vi "Prime BSI R3 Get Set ROI.vi"(0 "Prime Notifier":refnum<notifier>, 7 "IDS Actions":T2, 11 "Camera Handle":u32, 13 "Image Ref":T1) -> (4 "Prime Notifier (Dup)":refnum<notifier>, 15 "Error":errorcluster)   [LabVIEW 2016]
uses:
  Prime Controls/Prime Notifier Element.ctl
  Prime Controls/Prime Actions.ctl
  Prime Controls/Prime Parameters.ctl
  Prime Controls/Prime Parameter List.ctl
  Prime Controls/Prime ROI.ctl
  <vilib>/vision/Image Controls.llb/IMAQ Image.ctl
  Prime Controls/Prime IMAQ Key Info.ctl
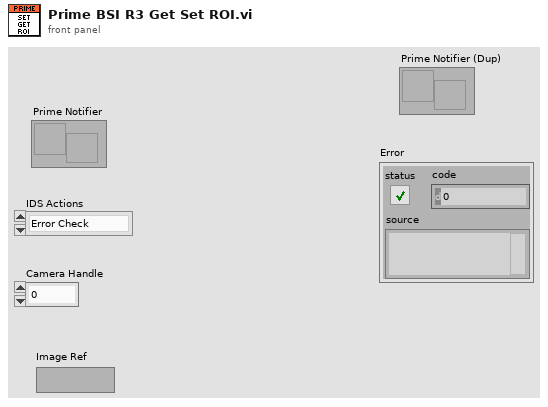
[diagram p1: front panel]
types:
  T1 = typedef "IMAQ Image.ctl" = refnum<image>
  T2 = typedef "Prime Actions.ctl" = enum16{"Error Check", "Initialize", "Preview", "Record", "Abort", "Record Settings", "Set Parameter", "Get Parameter", "Set ROI", "Get ROI", "Status", "Quit"}
  T3 = typedef "Prime IMAQ Key Info.ctl" = cluster{"Frame":u32, "Sensor Height":i32, "Sensor Width":i32, "ROI Height":i32, "ROI Width":i32, "ROI Enable?":bool, "Bit per Pixel":u8}
  T4 = typedef "Prime ROI.ctl" = cluster{"X Start":u32, "X End":u32, "X Bin":u32, "Y Start":u32, "Y End":u32, "Y Bin":u32}
  T5 = typedef "Prime Notifier Element.ctl" = cluster{"Prime Actions":T2, "Received?":bool, "Prime Parameter":T6, "Prime ROI":T4, "Running?":bool, "File Path":path, "# of frames":i32, "Image Ref":T1, "Error":errorcluster}
  T6 = typedef "Prime Parameters.ctl" = cluster{"Parameter":T7, "Value":dbl}
  T7 = typedef "Prime Parameter List.ctl" = enum16{"Exposure Time (s)"}
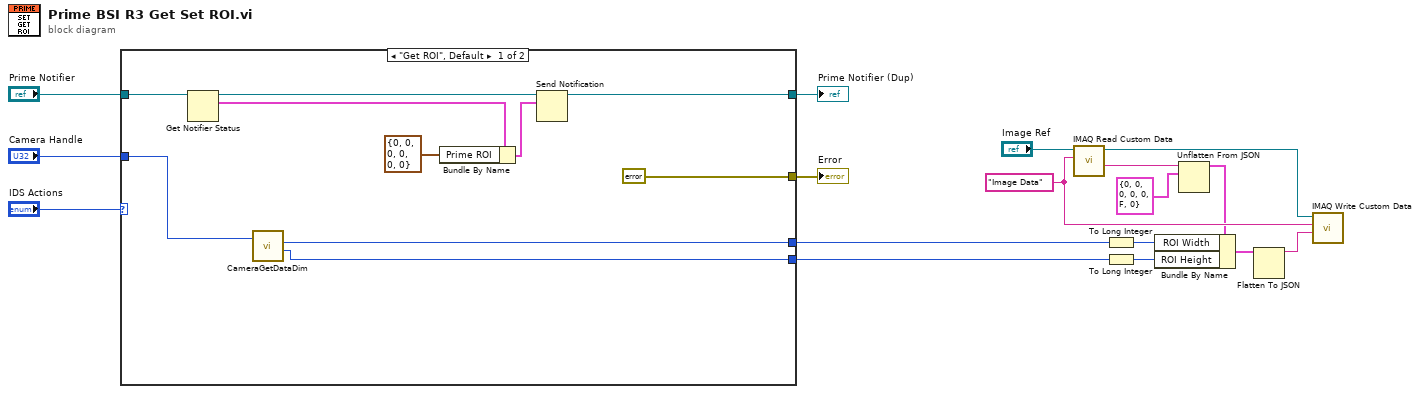
[diagram p0: block diagram]
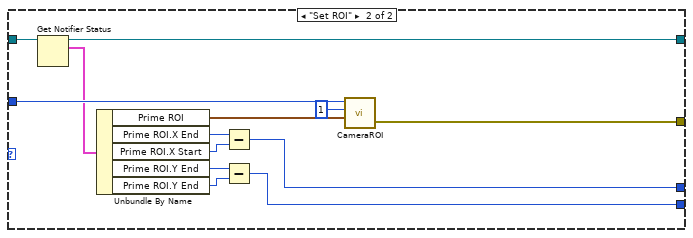
[diagram p2: hidden frame]
diagram:
  w12 = "Image Data" ("Key")
  n1 = case shown="\"Get ROI\", Default" "IDS Actions" {
    tunnel: "Prime Notifier" -> [w27 w38]
    tunnel: [w25 w37] -> w15
    tunnel: "Camera Handle" -> [w20 w40]
    tunnel: [errorcluster {"status"=FALSE, "code"=0, "source"=""} ("error out") w34] -> w13
    tunnel: [w19 w29] -> w1
    tunnel: [w18 w28] -> w2
    frame "Get ROI", Default {
      n2 = Get Notifier Status(notifier=w27) -> (notifier out=w26:refnum<notifier>, current notification=w24:T5)  [unwired: 1 in, 3 out]
      n3 = call <userlib>:"CameraGetDataDim.vi"("Camera Handle"=w20) -> ("Xdim"=w19:u32, "Ydim"=w18:u32)  [unwired: 1 in, 2 out]
      n4 = Bundle By Name(cluster=w24, "Prime ROI"=T4 {"X Start"=0, "X End"=0, "X Bin"=0, "Y Start"=0, "Y End"=0, "Y Bin"=0} ("IDS ROI")) -> (w23:T5)
      n5 = Send Notification(notification=w23, notifier=w26) -> (notifier out=w25:refnum<notifier>)  [unwired: 1 in, 1 out]
    }
    frame "Set ROI" {
      n6 = Get Notifier Status(notifier=w38) -> (notifier out=w37:refnum<notifier>, current notification=w36:T5)  [unwired: 1 in, 3 out]
      n7 = Unbundle By Name(w36) -> ("Prime ROI"=w35:T4, "Prime ROI.X End"=w33:u32, "Prime ROI.X Start"=w32:u32, "Prime ROI.Y End"=w31:u32, "Prime ROI.Y End"=w30:u32)
      n8 = Subtract(x=w33, y=w32) -> (x-y=w29:u32)
      n9 = Subtract(x=w31, y=w30) -> (x-y=w28:u32)
      n10 = call <userlib>:"CameraROI.vi"("ROI Params"=w35, "ROI Index"=u32 1, "Camera Handle"=w40) -> ("error out"=w34:errorcluster)  [unwired: 1 in, 1 out]
    }
  }
  "Error" <- w13
  "Prime Notifier (Dup)" <- w15
  n11 = call "IMAQ Read Custom Data"("Key"=w12, "Image"="Image Ref") -> ("Custom Data Out"=w5:string, "Image (duplicate)"=w4:T1)  [unwired: 7 in, 1 out]
  n12 = To Long Integer(number=w1) -> (32bit integer=w10:i32)
  n13 = To Long Integer(number=w2) -> (32bit integer=w11:i32)
  n14 = Unflatten From JSON(JSON string=w5, type and defaults=T3 {"Frame"=0, "Sensor Height"=0, "Sensor Width"=0, "ROI Height"=0, "ROI Width"=0, "ROI Enable?"=FALSE, "Bit per Pixel"=0} ("IDS IMAQ Key Info")) -> (value=w6:T3)  [unwired: 5 in, 1 out]
  n15 = Bundle By Name(cluster=w6, "ROI Width"=w10, "ROI Height"=w11) -> (w8:T3)
  n16 = Flatten To JSON(anything=w8) -> (JSON string=w9:string)  [unwired: 2 in, 1 out]
  n17 = call "IMAQ Write Custom Data"("Custom Data In"=w9, "Key"=w12, "Image"=w4) -> ()  [unwired: 7 in, 2 out]
